vi "set_table.vi"(8 "error in (no error)":errorcluster, 9 "Table":refnum<class "Table.lvclass">, 10 "table_name":string, 11 "Doc in":refnum<class "Doc.lvclass">) -> (0 "error out":errorcluster, 3 "Doc out":refnum<class "Doc.lvclass">)   [LabVIEW 2020, in "toml_edit.lvlib" / "Doc.lvclass"]
uses:
  Doc.lvclass
  Doc.lvclass/Doc.ctl
  Table/Table.lvclass
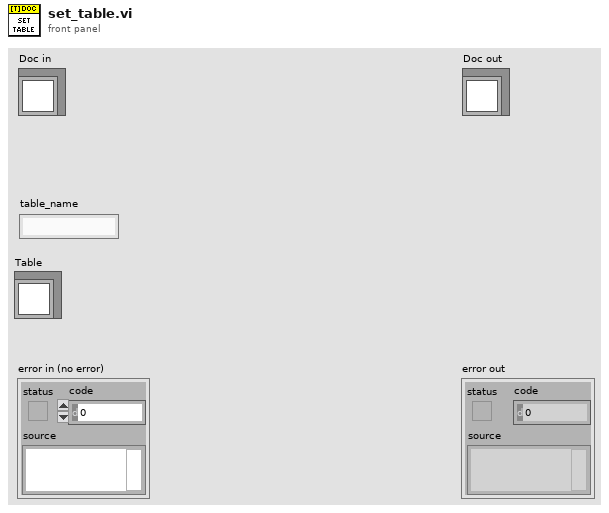
[diagram p1: front panel]
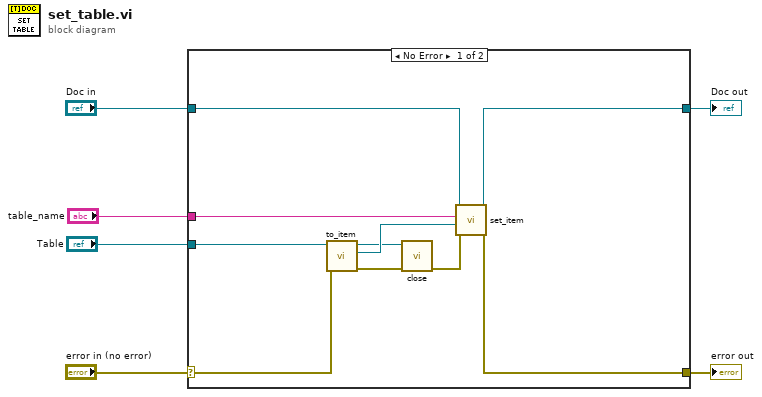
[diagram p0: block diagram]
diagram:
  n1 = case shown="No Error" "error in (no error)" {
    selector: "error in (no error)" -> [w10 w18]
    tunnel: [w9 w18] -> w5
    tunnel: [w8 w17] -> w3
    tunnel: "Doc in" -> [w7 w17]
    tunnel: "table_name" -> [w11 _]
    tunnel: "Table" -> [w12 _]
    frame No Error {
      n2 = call "to_item.vi"("error in (no error)"=w10, "Table in"=w12) -> ("error out"=w14:errorcluster, "Item out"=w16:refnum<class "Item.lvclass">, "Table out"=w15:refnum<class "Table.lvclass">)  [unwired: 7 in]
      n3 = call "close.vi"("error in (no error)"=w14, "Table in"=w15) -> ("error out"=w13:errorcluster)  [unwired: 9 in]
      n4 = call "set_item.vi"("error in (no error)"=w13, "Item"=w16, "item_name"=w11, "Doc in"=w7) -> ("error out"=w9:errorcluster, "Doc out"=w8:refnum<class "Doc.lvclass">)  [unwired: 6 in]
    }
    frame Error {
    }
  }
  "error out" <- w5
  "Doc out" <- w3
